vi "模式二.vi"() -> ()   [LabVIEW 2014]
panel:
  out "說明":string="本專題參考常見高中物理題型以及HW4。\n有一架轟炸機與一汽車水平距離為S0，轟炸機距離與地面維持高度H並保持固定速度Va水平飛行，汽車速度固定為Vc，請問轟炸機飛行多久後投彈可以命中汽車?Va、Vc、S0、H皆為變數，重力加速度為9.81，本程式會將時間點算出，並以動態圖示意。"
  out "車車":T1=TRUE
  out "合格":bool
  out "投彈時間(正解)":dbl
  in  "stop":bool
  in  "OK":bool
  in  "投彈時間(k)":dbl
  out "Va":dbl=120.0
  out "Vc":dbl=30.0
  out "H":dbl=122.5
  out "S0":i32=630
  out "轟炸機":T2=TRUE
  out "String":string
  out "炸彈":T3=TRUE
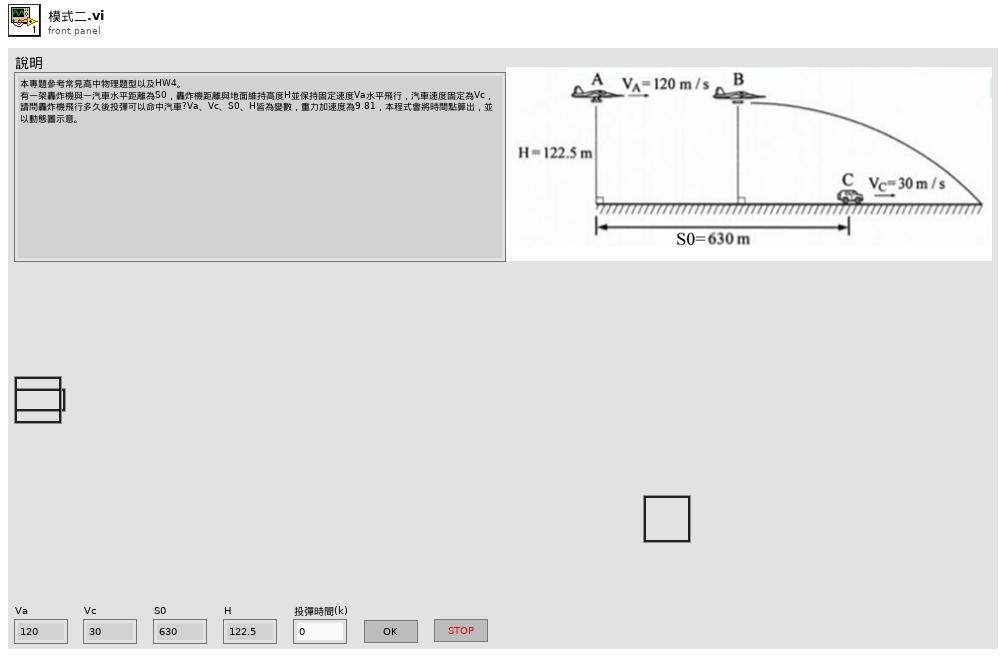
[diagram p1: front panel]
types:
  T1 = typedef "車!!.ctl" = bool
  T2 = typedef "飛機.ctl" = bool
  T3 = typedef "炸彈.ctl" = bool
  T4 = enum8{"Enabled", "Disabled", "Disabled and Grayed Out"}
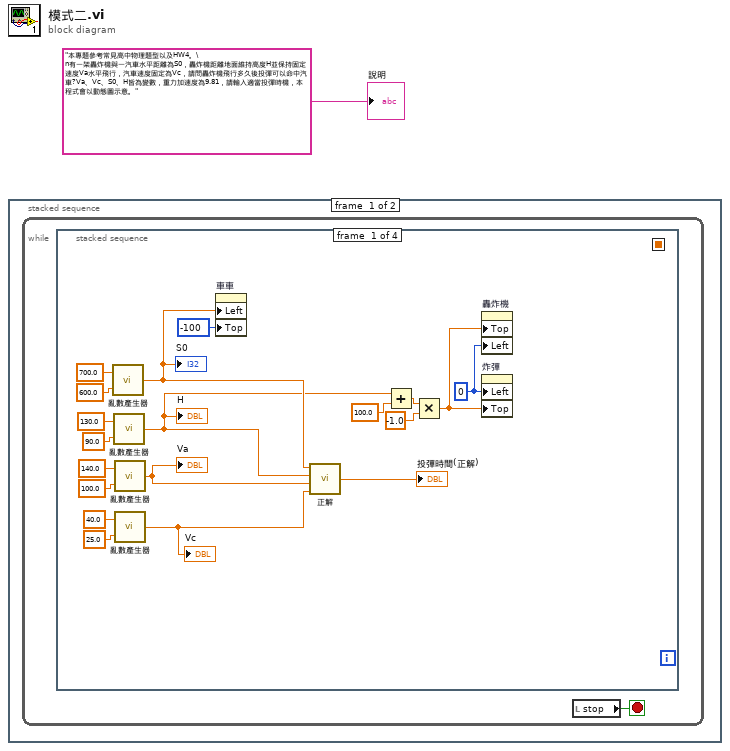
[diagram p0: block diagram]
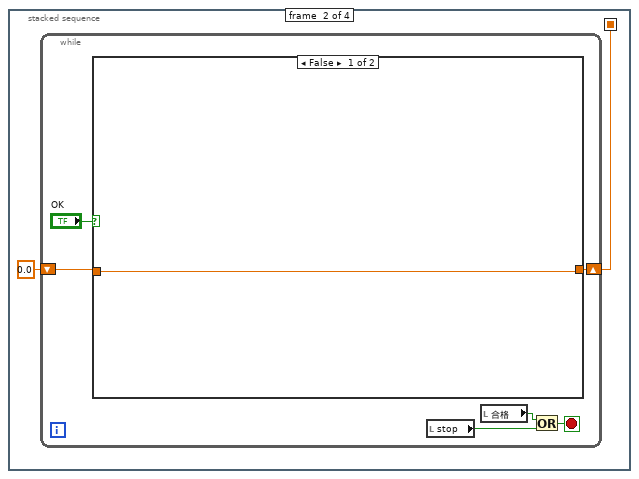
[diagram p2: hidden frame]
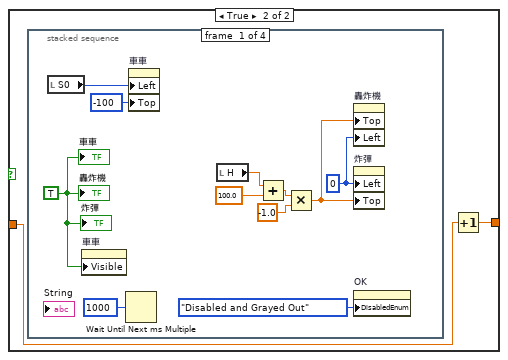
[diagram p3: hidden frame]
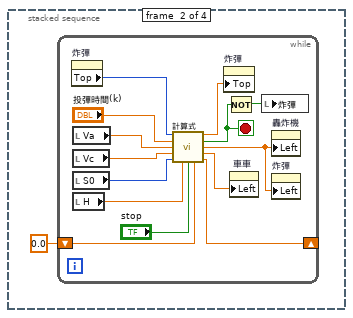
[diagram p4: hidden frame]
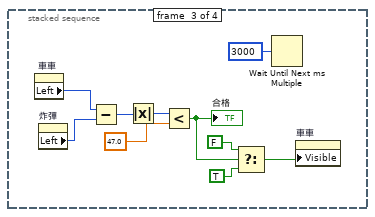
[diagram p5: hidden frame]
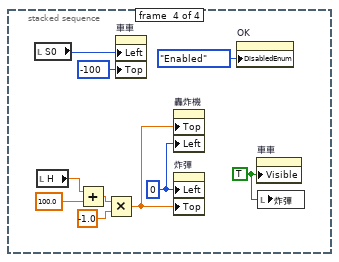
[diagram p6: hidden frame]
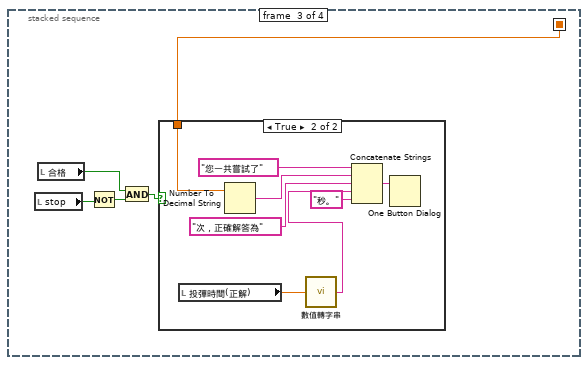
[diagram p7: hidden frame]
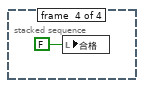
[diagram p9: hidden frame]
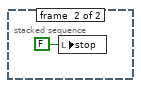
[diagram p10: hidden frame]
diagram:
  n1 = stacked-sequence {
    frame #0 {
      n2 = while {
        stop <- w2 stop-if-true
        n3 = stacked-sequence {
          seq-local: [_ w22 _ _] -> [_ _ w83 _]
          frame #0 {
            w6 = 0 ("Position:Left")
            n4 = call "亂數產生器.vi"("Min"=600.0, "Max"=700.0) -> ("Random"=w4:dbl)
            "S0" <- w4
            n5 = call "亂數產生器.vi"("Min"=90.0, "Max"=130.0) -> ("Random"=w3:dbl)
            "H" <- w3
            n6 = call "亂數產生器.vi"("Min"=100.0, "Max"=140.0) -> ("Random"=w12:dbl)
            "Va" <- w12
            n7 = call "亂數產生器.vi"("Min"=25.0, "Max"=40.0) -> ("Random"=w11:dbl)
            "Vc" <- w11
            n8 = property on="車車" class="Bool (strict)"("Left"=w4, "Top"=-100 ("Position:Top")) -> ()  [unwired: 2 in, 2 out]
            n9 = call "正解.vi"("Vc"=w11, "Va"=w12, "H"=w3, "S0"=w4) -> ("投彈時間(k)"=→"投彈時間(正解)":dbl)
            n10 = Add(x=w3, y=100.0) -> (x+y=w8:dbl)
            n11 = Multiply(x=w8, y=-1.0) -> (x*y=w7:dbl)
            n12 = property on="轟炸機" class="Bool (strict)"("Top"=w7, "Left"=w6) -> ()  [unwired: 2 in, 2 out]
            n13 = property on="炸彈" class="Bool (strict)"("Left"=w6, "Top"=w7) -> ()  [unwired: 2 in, 2 out]
          }
          frame #1 {
            n14 = while {
              shift-right: [w28] -> w22
              shift-left: 0.0 -> [w27]
              stop <- w24 stop-if-true
              n15 = case shown="False" "OK" {
                tunnel: w27 -> [w30 w32]
                tunnel: [w30 w31] -> w28
                frame False {
                }
                frame True {
                  n16 = stacked-sequence {
                    frame #0 {
                      w36 = 0 ("Position:Left")
                      w33 = TRUE
                      n17 = local read "S0"() -> (w42:i32)
                      n18 = property on="車車" class="Bool (strict)"("Visible"=w33) -> ()  [unwired: 2 in, 2 out]
                      n19 = Wait Until Next ms Multiple(millisecond multiple=u32 1000) -> ()  [unwired: 1 out]
                      n20 = property on="車車" class="Bool (strict)"("Left"=w42, "Top"=-100 ("Position:Top")) -> ()  [unwired: 2 in, 2 out]
                      n21 = local read "H"() -> (w34:dbl)
                      n22 = Add(x=w34, y=100.0) -> (x+y=w38:dbl)
                      n23 = Multiply(x=w38, y=-1.0) -> (x*y=w37:dbl)
                      n24 = property on="轟炸機" class="Bool (strict)"("Top"=w37, "Left"=w36) -> ()  [unwired: 2 in, 2 out]
                      n25 = property on="炸彈" class="Bool (strict)"("Left"=w36, "Top"=w37) -> ()  [unwired: 2 in, 2 out]
                      n26 = property on="OK" class="Bool"("DisabledEnum"=T4."Disabled and Grayed Out" ("Disabled")) -> ()  [unwired: 2 in, 2 out]
                      "車車" <- w33
                      "轟炸機" <- w33
                      "炸彈" <- w33
                    }
                    frame #1 {
                      n27 = while {
                        shift-right: [w49] -> _
                        shift-left: 0.0 -> [w53]
                        stop <- w46 stop-if-true
                        n28 = property on="炸彈" class="Bool (strict)"() -> ("Top"=w58:i32)  [unwired: 2 in, 2 out]
                        n29 = local read "Va"() -> (w57:dbl)
                        n30 = local read "Vc"() -> (w56:dbl)
                        n31 = local read "S0"() -> (w55:i32)
                        n32 = local read "H"() -> (w54:dbl)
                        n33 = call "計算式.vi"("b y"=w58, "投彈時間(k)"="投彈時間(k)", "Va"=w57, "Vc"=w56, "S0"=w55, "H"=w54, "stop"="stop", "ti"=w53) -> ("b y 2"=w52:dbl, "output stop"=w46:bool, "a x"=w51:dbl, "c x"=w50:dbl, "to"=w49:dbl)  [unwired: 3 in]
                        n34 = property on="炸彈" class="Bool (strict)"("Top"=w52) -> ()  [unwired: 2 in, 2 out]
                        n35 = Not(x=w46) -> (.not. x?=w45:bool)
                        n36 = property on="車車" class="Bool (strict)"("Left"=w50) -> ()  [unwired: 2 in, 2 out]
                        n37 = local write "炸彈"(w45) -> ()
                        n38 = property on="轟炸機" class="Bool (strict)"("Left"=w51) -> ()  [unwired: 2 in, 2 out]
                        n39 = property on="炸彈" class="Bool (strict)"("Left"=w51) -> ()  [unwired: 2 in, 2 out]
                      }
                    }
                    frame #2 {
                      n40 = property on="車車" class="Bool (strict)"() -> ("Left"=w64:i32)  [unwired: 2 in, 2 out]
                      n41 = property on="炸彈" class="Bool (strict)"() -> ("Left"=w68:i32)  [unwired: 2 in, 2 out]
                      n42 = Subtract(x=w64, y=w68) -> (x-y=w67:i32)
                      n43 = Absolute Value(x=w67) -> (abs(x)=w66:i32)
                      n44 = Less?(x=w66, y=47.0) -> (x < y?=w63:bool)
                      "合格" <- w63
                      n45 = Select(t=FALSE, s=w63, f=TRUE) -> (s? t:f=w62:bool)
                      n46 = Wait Until Next ms Multiple(millisecond multiple=u32 3000) -> ()  [unwired: 1 out]
                      n47 = property on="車車" class="Bool (strict)"("Visible"=w62) -> ()  [unwired: 2 in, 2 out]
                    }
                    frame #3 {
                      w69 = TRUE ("Visible")
                      w72 = 0 ("Position:Left")
                      n48 = local read "S0"() -> (w76:i32)
                      n49 = local read "H"() -> (w70:dbl)
                      n50 = Add(x=w70, y=100.0) -> (x+y=w74:dbl)
                      n51 = Multiply(x=w74, y=-1.0) -> (x*y=w73:dbl)
                      n52 = property on="車車" class="Bool (strict)"("Left"=w76, "Top"=-100 ("Position:Top")) -> ()  [unwired: 2 in, 2 out]
                      n53 = property on="轟炸機" class="Bool (strict)"("Top"=w73, "Left"=w72) -> ()  [unwired: 2 in, 2 out]
                      n54 = property on="炸彈" class="Bool (strict)"("Left"=w72, "Top"=w73) -> ()  [unwired: 2 in, 2 out]
                      n55 = property on="OK" class="Bool"("DisabledEnum"=T4."Enabled" ("Disabled")) -> ()  [unwired: 2 in, 2 out]
                      n56 = property on="車車" class="Bool (strict)"("Visible"=w69) -> ()  [unwired: 2 in, 2 out]
                      n57 = local write "炸彈"(w69) -> ()
                    }
                  }
                  n58 = Increment(x=w32) -> (x+1=w31:dbl)
                }
              }
              n59 = local read "stop"() -> (w25:bool)
              n60 = local read "合格"() -> (w26:bool)
              n61 = Or(x=w26, y=w25) -> (x .or. y?=w24:bool)
            }
          }
          frame #2 {
            n62 = local read "stop"() -> (w82:bool)
            n63 = local read "合格"() -> (w79:bool)
            n64 = Not(x=w82) -> (.not. x?=w80:bool)
            n65 = And(x=w79, y=w80) -> (x .and. y?=w81:bool)
            n66 = case shown="True" w81 {
              tunnel: w83 -> [_ w87]
              frame False {
              }
              frame True {
                n67 = local read "投彈時間(正解)"() -> (w86:dbl)
                n68 = Number To Decimal String(number=w87) -> (decimal integer string=w89:string)  [unwired: 1 in]
                n69 = call "數值轉字串.vi"("number"=w86) -> ("s? t:f"=w85:string)
                n70 = Concatenate Strings("您一共嘗試了" ("string"), w89, "次，正確解答為" ("string"), w85, "秒。" ("string")) -> (w91:string)
                n71 = One Button Dialog(message=w91) -> ()  [unwired: 1 in, 1 out]
              }
            }
          }
          frame #3 {
            n72 = local write "合格"(FALSE) -> ()
          }
        }
        n73 = local read "stop"() -> (w2:bool)
      }
    }
    frame #1 {
      n74 = local write "stop"(FALSE ("stop")) -> ()
    }
  }
  "說明" <- "本專題參考常見高中物理題型以及HW4。\n有一架轟炸機與一汽車水平距離為S0，轟炸機距離地面維持高度H並保持固定速度Va水平飛行，汽車速度固定為Vc，請問轟炸機飛行多久後投彈可以命中汽車?Va、Vc、S0、H皆為變數，重力加速度為9.81，請輸入適當投彈時機，本程式會以動態圖示意。" ("說明")
